vi "Open.vi"(8 "ErrorIn":errorcluster, 9 "StartupConfiguration":string, 11 "ReferenceIn":refnum<class "IApplicationConfiguration.lvclass">) -> (0 "ErrorOut":errorcluster, 3 "ReferenceOut":refnum<class "IApplicationConfiguration.lvclass">)   [LabVIEW 2021, in "IApplicationConfiguration.lvclass"]
uses:
  IApplicationConfiguration.lvclass
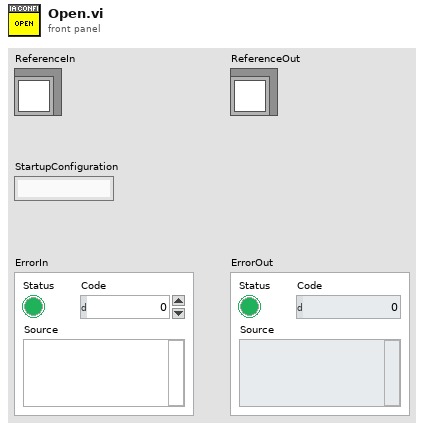
[diagram p1: front panel]
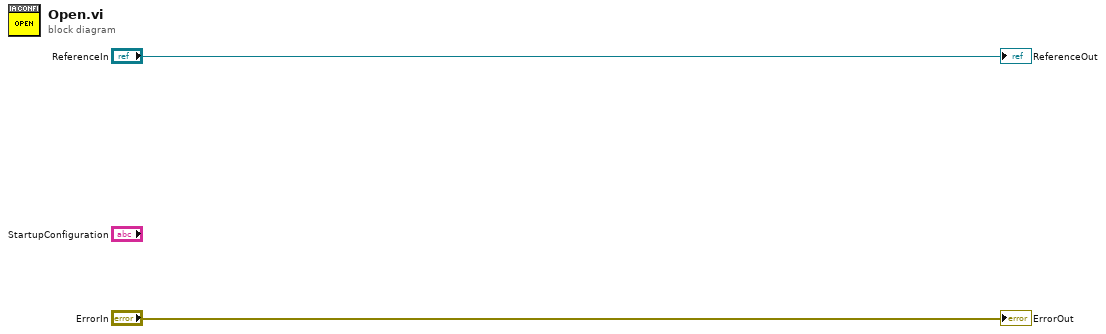
[diagram p0: block diagram]
diagram:
  "ErrorOut" <- "ErrorIn"
  "ReferenceOut" <- "ReferenceIn"
